vi "ReadStr.vi"(8 "error in":errorcluster caption="错误输入（无错误）", 9 "路径":string="data\\data.ini", 11 "section":string caption="Section") -> (0 "error out":errorcluster caption="错误输出", 1 "ConfigPath":string, 3 "Value":string[](array[string]))   [LabVIEW 2013]
uses:
  <vilib>/Utility/config.llb/Read Key (String).vi
  <vilib>/Utility/config.llb/NI_LVConfig.lvlib
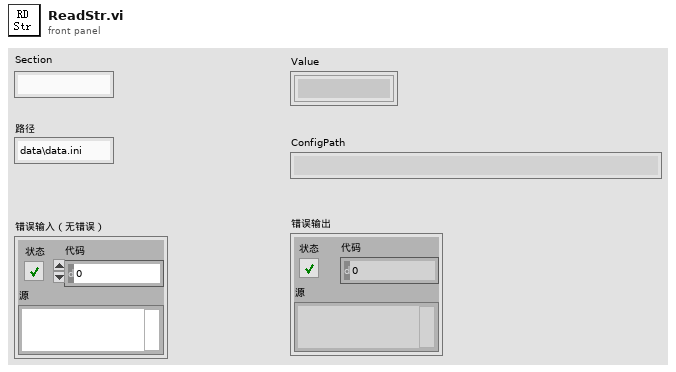
[diagram p1: front panel]
types:
  T1 = enum32{"invalid app kind", "Development System", "Run Time System", "Student Edition", "Embedded LabVIEW", "Evaluation", "Custom"}
  T2 = typedef "NI_LVConfig.lvlib/Config Data RefNum.ctl" = refnum<k1>
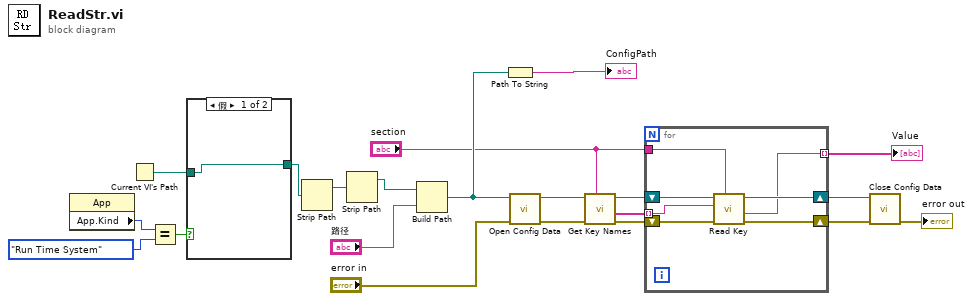
[diagram p0: block diagram]
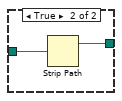
[diagram p2: hidden frame]
diagram:
  n1 = property class="App"() -> ("App.Kind"=w21:T1)  [unwired: 2 in, 2 out]
  n2 = Current VI's Path() -> (path=w18:path)
  n3 = Equal?(x=w21, y=T1."Run Time System" ("应用程序:类别")) -> (x = y?=w19:bool)
  n4 = case shown="假" w19 {
    tunnel: w18 -> [w22 w24]
    tunnel: [w22 w23] -> w17
    frame False {
    }
    frame True {
      n5 = Strip Path(path=w24) -> (stripped path=w23:path)  [unwired: 1 out]
    }
  }
  n6 = Strip Path(path=w17) -> (stripped path=w16:path)  [unwired: 1 out]
  n7 = Strip Path(path=w16) -> (stripped path=w1:path)  [unwired: 1 out]
  n8 = Build Path(base path=w1, name or relative path="路径") -> (appended path=w12:path)
  n9 = Path To String(path=w12) -> (string=→"ConfigPath":string)
  n10 = call <vilib>:"Open Config Data.vi"("error in (no error)"="error in", "configuration file path"=w12) -> ("error out"=w10:errorcluster, "refnum"=w11:T2)  [unwired: 7 in, 1 out]
  n11 = call <vilib>:"Get Key Names.vi"("section"="section", "error in (no error)"=w10, "refnum"=w11) -> ("error out"=w8:errorcluster, "key names"=w7:string[], "refnum out"=w9:T2)  [unwired: 5 in, 1 out]
  n12 = for {
    shift-right: [w27] -> w4
    shift-left: w9 -> [w31]
    shift-right: [w26] -> w3
    shift-left: w8 -> [w28]
    tunnel: w7 -> [w30] mode=indexing
    tunnel: "section" -> [w29]
    tunnel: [w25] -> w5 mode=indexing
    n13 = call-poly <vilib>:"Read Key.vi"("section"=w29, "error in (no error)"=w28, "key"=w30, "refnum"=w31) -> ("error out"=w26:errorcluster, "value"=w25:string, "refnum out"=w27:T2)  [unwired: 4 in, 1 out]
  }
  "Value" <- w5
  n14 = call <vilib>:"Close Config Data.vi"("error in (no error)"=w3, "refnum"=w4) -> ("error out"=→"error out":errorcluster)  [unwired: 8 in, 1 out]
